vi "Convert ASCII to Unicode.vi"(11 "ASCII":string="Hello World") -> (3 "Unicode":string)   [LabVIEW 2019]
uses:
  <vilib>/addons/Tools/Unicode/UI Unicode Tools.lvlib
panel:
  out "Unicode displayed on an ASCII indicator":string
  out "ASCII (hex)":string
  out "Unicode (hex)":string
  out "ASCII (hex)":string
  out "ASCII":string
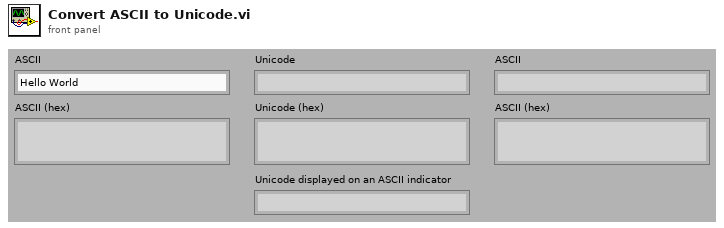
[diagram p1: front panel]
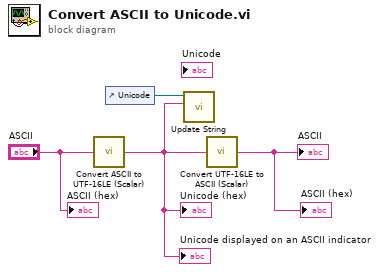
[diagram p0: block diagram]
diagram:
  n1 = call <vilib>:"Convert ASCII to UTF-16LE (Scalar).vi"("ASCII"="ASCII") -> ("Unicode"=w1:string)  [unwired: 4 in]
  "Unicode (hex)" <- w1
  "Unicode displayed on an ASCII indicator" <- w1
  n2 = control-ref of="Unicode"() -> (w2:refnum<vi>)
  n3 = call <vilib>:"Update String.vi"("String Value"=w1, "String Control Reference"=w2) -> ()  [unwired: 6 in, 2 out]
  n4 = call <vilib>:"Convert UTF-16LE to ASCII (Scalar).vi"("Unicode"=w1) -> ("ASCII"=→"ASCII" →"ASCII (hex)":string)  [unwired: 4 in]
  "ASCII (hex)" <- "ASCII"
